vi "Vector x A (Optimized).vi"(2 "Matrix A":T1, 3 "Vector V'":dbl[](array[numeric])) -> (0 "error":i32, 1 "V' x A":dbl[](array[numeric]))   [LabVIEW 2017, in "NI_AALBase.lvlib"]
uses:
  NI_AALBase.lvlib
  RealMatrix.ctl
  <resource>/lvanlys.dll
  NI_Matrix.lvlib
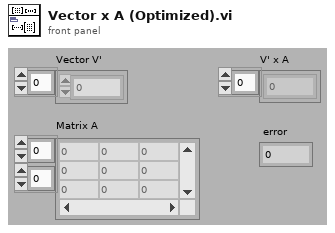
[diagram p1: front panel]
types:
  T1 = typedef "NI_Matrix.lvlib/RealMatrix.ctl" = dbl[][]
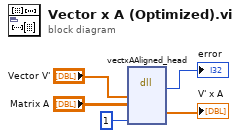
[diagram p0: block diagram]
diagram:
  n1 = dll-call lib="C:/Program Files (x86)/National Instruments/LabVIEW 2017/resource/lvanlys.*" fn="vectxAAligned_head"("xHandle"="Vector V'", "aHandle"="Matrix A", "isAligned"=1) -> ("return type"=→"error":i32, "yHandle"=→"V' x A":dbl[])  [unwired: 7 in, 2 out]
